vi "ort_fit_calcIntermediate.vi"(8 "inputValid":bool, 11 "ort.fit.p.params":T2) -> (2 "paramExtractDebug":cluster{"index":u16, "minimum":i16}, 3 "output cluster":T1)   [LabVIEW 2016]
uses:
  <vilib>/rvi/Emulation/niFpgaEmulationIsFPGAContextNoSignature.vi
  <vilib>/rvi/DataTransferAndStorage/Container/Common/niFpgaContainerGetUniqueNameForEmu.vi
  <vilib>/rvi/eio/common/nirviEmuReportErrorAndStop.vi
  <vilib>/rvi/Emulation/niFpgaSctlEmulationGetInTimedLoop.vi
  <vilib>/rvi/Emulation/niFpgaProcessEmulError.vi
  <vilib>/rvi/Memory/Memory_Emulation/niFpgaMemoryEmulationCacheClearOnFirstRun.vi
  <vilib>/rvi/Memory/Memory_Emulation/nirvimemoryEmulationManagerCache_MakeExclusive.vi
  <vilib>/rvi/Memory/Memory_Emulation/niFpgaMemoryEmulationValidateCache.vi
  <vilib>/rvi/Memory/Memory_Emulation/nirvimemoryEmulationManagerCache_InsertValue.vi
  <vilib>/Utility/error.llb/Clear Errors.vi
  <vilib>/rvi/Memory/Memory_Emulation/nirvimemoryEmulationManagerCache_ReleaseExclusive.vi
  <vilib>/rvi/Memory/Memory_Emulation/nirvimemoryEmulationManagerCache_GetValue.vi
  <vilib>/rvi/Memory/Memory_Emulation/nirvimemoryEmulationManagerCache_SetValue.vi
  <vilib>/rvi/errors/niFpgaSetErrorForExecOnDevCompSimple.vi
  <vilib>/rvi/FIFO/Fifo_Resource/nirvififoEmulationSetSize.vi
  <vilib>/rvi/FIFO/Fifo_Resource/nirviFifoEmulationQueueMgr.vi
  <instcachedir>/0/nirviFifoEmulationQueueMgr_E5CAEC123FF24DC58D834DCA3CDAA9B5.lvgen/nirviFifoEmulationQueueMgr_E5CAEC123FF24DC58D834DCA3CDAA9B5_002.vi
  <vilib>/rvi/FIFO/Fifo_Resource/nirvififoEmulationDetermineInputValidOut.vi
  <vilib>/rvi/FIFO/Fifo_Resource/nirvififoEmulationCreateLock.vi
  <vilib>/rvi/FIFO/Fifo_Resource/nirvififoEmulationObtainLock.vi
  <vilib>/rvi/FIFO/Fifo_Resource/nirvififoEmulationReleaseLock.vi
  <vilib>/rvi/occurrence/nirviWaitOnOccurrenceBase.vi
  <vilib>/rvi/errors/nirviReportUnexpectedCaseInternalError.vi
  <vilib>/rvi/errors/nirviReportUnexpectedCaseInternalError (U32).vi
  <instcachedir>/0/nirviFifoEmulationQueueMgr_E5CAEC123FF24DC58D834DCA3CDAA9B5.lvgen/nirviFifoEmulationQueueMgr_E5CAEC123FF24DC58D834DCA3CDAA9B5_001.vi
  <instcachedir>/0/nirviFifoEmulationQueueMgr_E5CAEC123FF24DC58D834DCA3CDAA9B5.lvgen/nirviFifoEmulationQueueMgr_E5CAEC123FF24DC58D834DCA3CDAA9B5_007.vi
  <vilib>/rvi/DataTransferAndStorage/Container/XNode/niFpgaContainer.xnode
  <vilib>/rvi/DataTransferAndStorage/Handshake/Emulation/niFpgaHandshakeEmulation.vi
  <vilib>/rvi/DataTransferAndStorage/Register/Emulation/niFpgaRegisterEmulation.vi
  <vilib>/rvi/FIFO/Fifo_Resource/nirvififoEmulationWrite.vi
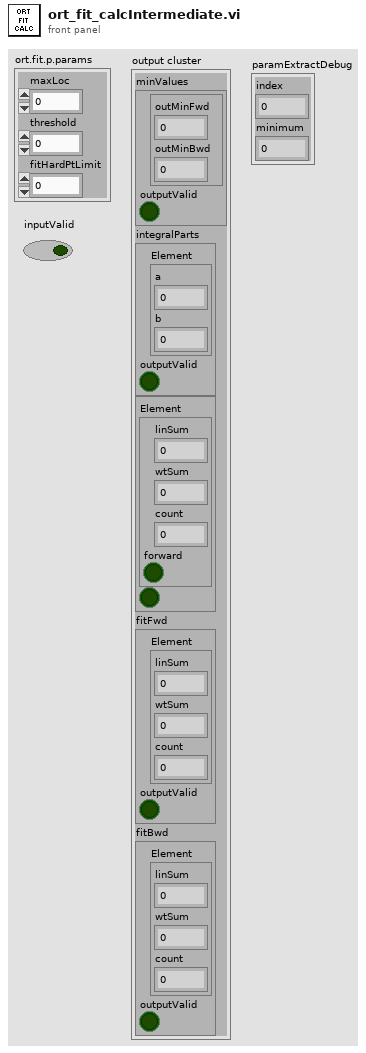
[diagram p1: front panel]
types:
  T1 = cluster{"minValues":cluster{cluster{"outMinFwd":fxp<+/-,22,1>, "outMinBwd":fxp<+/-,22,1>}, "outputValid":bool}, "integralParts":cluster{"Element":cluster{"a":i32, "b":i32}, "outputValid":bool}, cluster{"Element":cluster{"linSum":i32, "wtSum":fxp<+/-,54,34>, "count":u16, "forward":bool}, bool}, "fitFwd":cluster{"Element":cluster{"linSum":i32, "wtSum":fxp<+/-,54,34>, "count":u16}, "outputValid":bool}, "fitBwd":cluster{"Element":cluster{"linSum":i32, "wtSum":fxp<+/-,54,34>, "count":u16}, "outputValid":bool}}
  T2 = cluster{"maxLoc":u16, "threshold":i16, "fitHardPtLimit":u16}
  T3 = cluster{"linSum":i32, "wtSum":fxp<+/-,54,34>, "count":u16, "forward":bool}
  T4 = cluster{cluster{"outMinFwd":fxp<+/-,22,1>, "outMinBwd":fxp<+/-,22,1>}, "outputValid":bool}
  T5 = cluster{"Element":cluster{"a":i32, "b":i32}, "outputValid":bool}
  T6 = cluster{"Element":cluster{"linSum":i32, "wtSum":fxp<+/-,54,34>, "count":u16}, "outputValid":bool}
  T7 = cluster{"outMinFwd":fxp<+/-,22,1>, "outMinBwd":fxp<+/-,22,1>}
  T8 = cluster{"linSum":i32, "wtSum":fxp<+/-,54,34>, "count":u16}
  T9 = cluster{"Element":cluster{"linSum":i32, "wtSum":fxp<+/-,54,34>, "count":u16, "forward":bool}, bool}
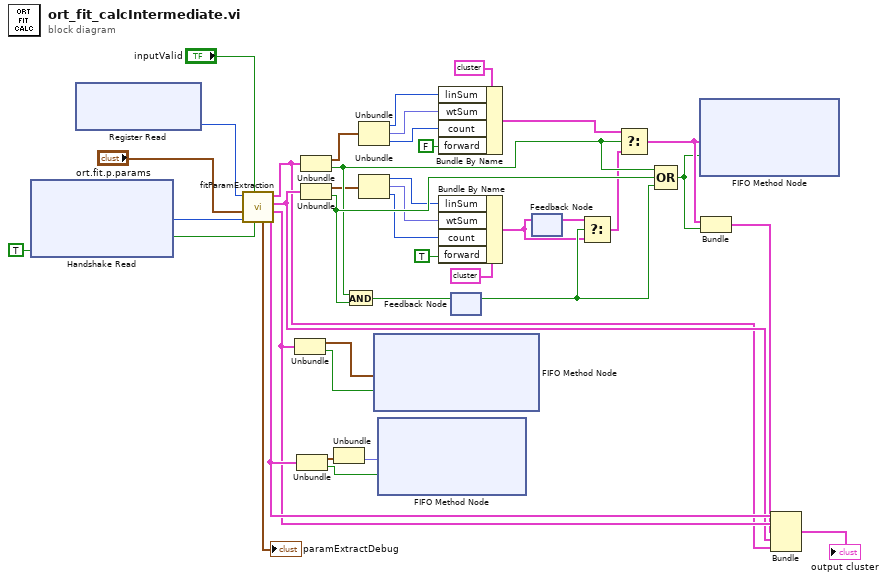
[diagram p0: block diagram]
diagram:
  n1 = xnode ("Handshake Read")("Ready for Output"=TRUE) -> ("Data"=w12:u16, "Output Valid"=w13:bool)  [unwired: 1 in, 1 out]
  n2 = xnode ("Register Read")() -> ("Data"=w40:u16)  [unwired: 1 in, 1 out]
  n3 = call "fitParamExtraction.vi"("startFit"=w13, "inputValid"="inputValid", "startIndex"=w12, "fittingParams"="ort.fit.p.params", "waveLength"=w40) -> ("minValues"=w10:T4, "integralParts"=w9:T5, "fitFwd"=w3:T6, "fitBwd"=w2:T6, "debugOut"=→"paramExtractDebug":cluster{"index":u16, "minimum":i16})  [unwired: 2 in]
  n4 = Unbundle(w9) -> ("Element"=w35:cluster{"a":i32, "b":i32}, "outputValid"=w36:bool)
  n5 = Unbundle(w10) -> (w37:T7, "outputValid"=w39:bool)
  n6 = Unbundle(w2) -> ("Element"=w16:T8, "outputValid"=w32:bool)
  n7 = Unbundle(w3) -> ("Element"=w22:T8, "outputValid"=w33:bool)
  n8 = Unbundle(w37) -> ("outMinBwd"=w38:fxp<+/-,22,1>)  [unwired: 1 out]
  n9 = And(x=w32, y=w33) -> (x .and. y?=w28:bool)
  n10 = Unbundle(w16) -> ("linSum"=w17:i32, "wtSum"=w18:fxp<+/-,54,34>, "count"=w19:u16)
  n11 = Unbundle(w22) -> ("linSum"=w25:i32, "wtSum"=w26:fxp<+/-,54,34>, "count"=w27:u16)
  n12 = xnode ("FIFO Method Node")("Element"=w35, "Input Valid"=w36) -> ()  [unwired: 1 in, 2 out]
  n13 = xnode ("FIFO Method Node")("Element"=w38, "Input Valid"=w39) -> ()  [unwired: 1 in, 2 out]
  n14 = Bundle By Name(cluster=T3 {"linSum"=0, "wtSum"=0.0, "count"=0, "forward"=FALSE} ("Element"), "linSum"=w17, "wtSum"=w18, "count"=w19, "forward"=FALSE) -> (w21:T3)
  n15 = Bundle By Name(cluster=T3 {"linSum"=0, "wtSum"=0.0, "count"=0, "forward"=FALSE} ("Element"), "linSum"=w25, "wtSum"=w26, "count"=w27, "forward"=TRUE) -> (w31:T3)
  n16 = feedback #1() -> (w34:bool)  [unwired: 1 in]
  n17 = feedback-in #1(w28) -> ()
  n18 = feedback #2() -> (w30:T3)  [unwired: 1 in]
  n19 = feedback-in #2(w31) -> ()
  n20 = Select(t=w30, s=w34, f=w31) -> (s? t:f=w29:T3)
  n21 = Select(t=w21, s=w32, f=w29) -> (s? t:f=w8:T3)
  n22 = Compound Arithmetic op=OR(w32, w33, w34) -> (w7:bool)
  n23 = xnode ("FIFO Method Node")("Element"=w8, "Input Valid"=w7) -> ()  [unwired: 1 in, 2 out]
  n24 = Bundle("Element"=w8, w7) -> (w6:T9)  [unwired: 1 in]
  n25 = Bundle("minValues"=w10, "integralParts"=w9, w6, "fitFwd"=w3, "fitBwd"=w2) -> (→"output cluster":T1)  [unwired: 1 in]
